vi "Get both currents.vi"(5 "error In":errorcluster, 6 "VI reference":refnum<vi>) -> (0 "error out":errorcluster, 1 "SC Current [kA]":dbl format="%.5f", 2 "Current [KA]":dbl format="%.5f", 3 "dup VI reference":refnum<vi>, 4 "Status":T1)   [LabVIEW 2020]
uses:
  Sub Controls/PS Status.ctl
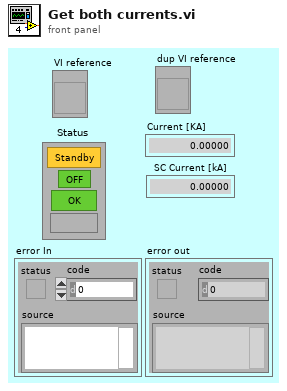
[diagram p1: front panel]
types:
  T1 = typedef "PS Status.ctl" = cluster{"PS On":bool, "PS Fault":bool, "Ramp Status":u16, "Cell Control":bool}
  T2 = cluster{"Current [KA]":dbl, "Current [KA] 2":dbl}
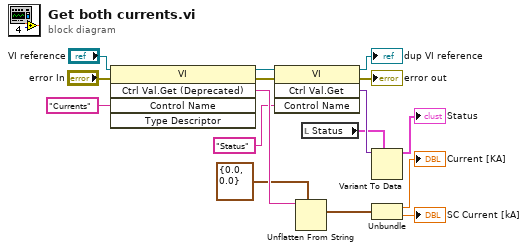
[diagram p0: block diagram]
diagram:
  n1 = invoke class="VI" method="Ctrl Val.Get (Deprecated)"(reference="VI reference", error in="error In", "Control Name"="Currents") -> (reference out=w6:refnum<vi>, error out=w8:errorcluster, "Get Control Value"=w14:string)  [unwired: 2 in, 2 out]
  n2 = invoke class="VI" method="Ctrl Val.Get"(reference=w6, error in=w8, "Control Name"="Status") -> (reference out=→"dup VI reference":refnum<vi>, error out=→"error out":errorcluster, "Get Control Value Variant"=w2:variant)  [unwired: 1 in, 1 out]
  n3 = Unflatten From String(type=T2 {"Current [KA]"=0.0, "Current [KA] 2"=0.0}, binary string=w14) -> (value=w11:T2)  [unwired: 3 in, 2 out]
  n4 = local read "Status"() -> (w1:T1)
  n5 = Variant To Data(type=w1, Variant=w2) -> (data=→"Status":T1)  [unwired: 1 in, 1 out]
  n6 = Unbundle(w11) -> ("Current [KA]"=→"Current [KA]":dbl, "Current [KA] 2"=→"SC Current [kA]":dbl)
